vi "Get Todo Bookmarks.vi"(6 "open VI references? (False)":bool, 8 "error in (no error)":errorcluster, 11 "Directory to Search":path) -> (0 "error out":errorcluster, 2 "todo bookmarks":map{path, T1}(c390), 3 "unreadable VIs (errors)":path[](array[path]))   [LabVIEW 2021]
uses:
  <vilib>/Utility/miscctls.llb/LVBookmarkInfoTypeDef.ctl
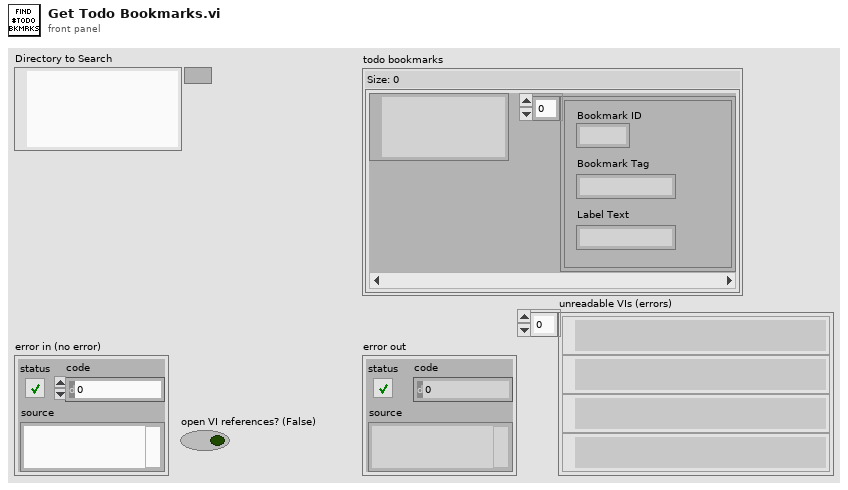
[diagram p1: front panel]
types:
  T1 = typedef "LVBookmarkInfoTypeDef.ctl" = cluster{"Bookmark ID":u32, "Bookmark Tag":string, "Label Text":string}[]
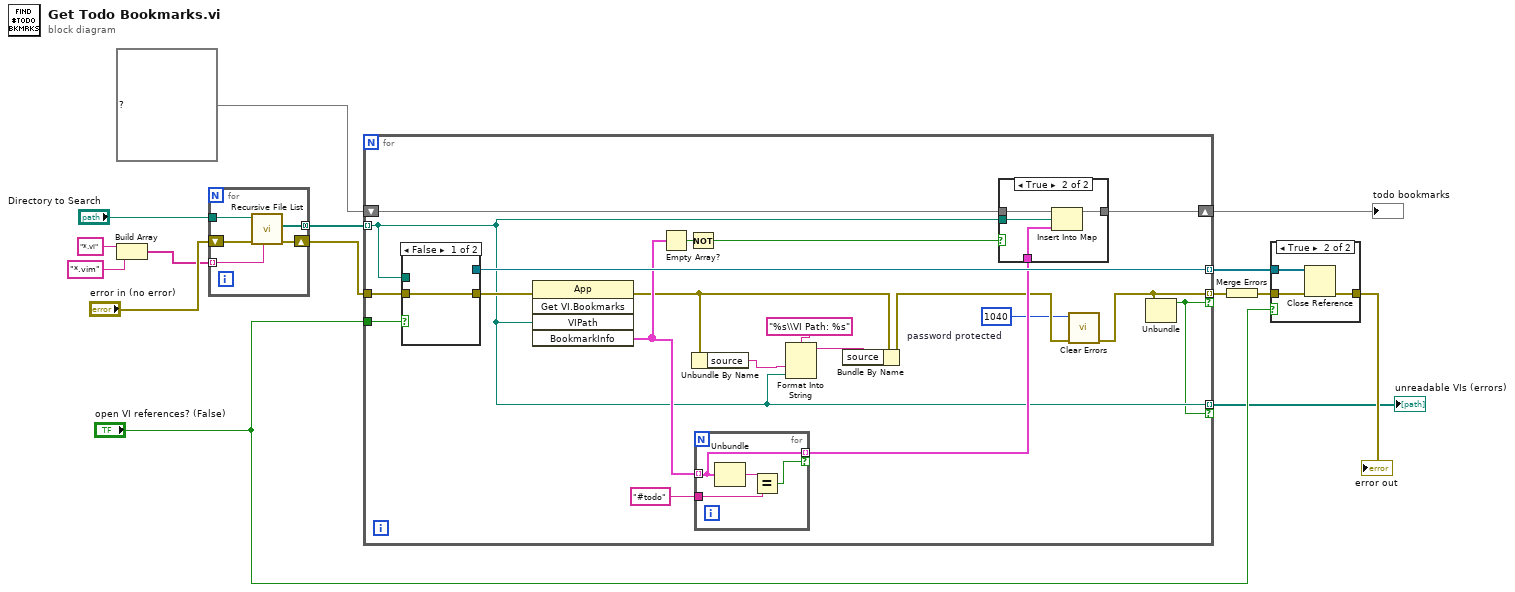
[diagram p0: block diagram]
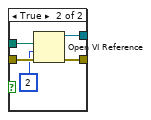
[diagram p3: hidden frame]
diagram:
  n1 = Build Array("*.vi" ("pattern"), "*.vim" ("pattern")) -> (w1:string[])
  n2 = for {
    tunnel: [w18] -> w8 mode=concatenating
    tunnel: w1 -> [w17] mode=indexing
    tunnel: "Directory to Search" -> [w16]
    shift-right: [w19] -> w13
    shift-left: "error in (no error)" -> [w20]
    n3 = call <vilib>:"Recursive File List.vi"("pattern"=w17, "error in (no error)"=w20, "Folder Path"=w16) -> ("error out"=w19:errorcluster, "All Files in Dir"=w18:path[])  [unwired: 4 in, 3 out]
  }
  n4 = for {
    tunnel: w8 -> [w25] mode=indexing
    tunnel: [w39] -> w9 mode=indexing
    shift-right: [w37] -> w15
    shift-left: map{path, T1} {} ("empty map") -> [w33]
    tunnel: w13 -> [w38]
    tunnel: [w22] -> w10 mode=indexing if=w24
    tunnel: "open VI references? (False)" -> [w30]
    tunnel: [w25] -> w4 mode=indexing if=w24
    w21 = 1040  # password protected
    n5 = case shown="False" w30 {
      tunnel: [w41 w46] -> w40
      tunnel: [_ w45] -> w39
      tunnel: w38 -> [w41 w44]
      tunnel: w25 -> [_ w42]
      frame False {
      }
      frame True {
        n6 = Open VI Reference(vi path=w42, options=2, error in (no error)=w44) -> (vi reference=w45:refnum<vi>, error out=w46:errorcluster)  [unwired: 3 in]
      }
    }
    n7 = invoke class="App" method="Get VI.Bookmarks"(error in=w40, "VIPath"=w25) -> (error out=w29:errorcluster, "BookmarkInfo"=w32:T1)  [unwired: 3 in, 3 out]
    n8 = Empty Array?(array=w32) -> (empty?=w36:bool)
    n9 = Not(x=w36) -> (.not. x?=w35:bool)
    n10 = Unbundle By Name(w29) -> ("source"=w28:string)
    n11 = for {
      tunnel: w32 -> [w48] mode=indexing
      tunnel: "#todo" ("Bookmark Tag") -> [w49]
      tunnel: [w48] -> w31 mode=indexing if=w47
      n12 = Unbundle(w48) -> ("Bookmark Tag"=w50:string)  [unwired: 2 out]
      n13 = Equal?(x=w50, y=w49) -> (x = y?=w47:bool)
    }
    n14 = Format Into String(format string="%s\\VI Path: %s", w28, w25) -> (resulting string=w26:string)  [unwired: 2 in, 1 out]
    n15 = Bundle By Name(cluster=w29, "source"=w26) -> (w23:errorcluster)
    n16 = case shown="True" w35 {
      tunnel: w33 -> [w51 w55]
      tunnel: [w51 w54] -> w37
      tunnel: w25 -> [_ w53]
      tunnel: w31 -> [_ w52]
      frame False {
      }
      frame True {
        n17 = Insert Into Map(map in=w55, key=w53, value=w52) -> (map out=w54:map{path, T1})  [unwired: 2 out]
      }
    }
    n18 = call <vilib>:"Clear Errors.vi"("error in (no error)"=w23, "specific error code to clear (0: all)"=w21) -> ("error out"=w22:errorcluster)  [unwired: 4 in, 1 out]
    n19 = Unbundle(w22) -> ("status"=w24:bool)  [unwired: 2 out]
  }
  "todo bookmarks" <- w15
  "unreadable VIs (errors)" <- w4
  n20 = Merge Errors(w10) -> (w12:errorcluster)
  n21 = case shown="True" "open VI references? (False)" {
    tunnel: w12 -> [w56 w59]
    tunnel: [w56 w58] -> w11
    tunnel: w9 -> [_ w57]
    frame False {
    }
    frame True {
      n22 = Close Reference(reference=w57, error in (no error)=w59) -> (error out=w58:errorcluster)
    }
  }
  "error out" <- w11
